vi "Trim Context.vi"(1 "Qualified Name":string) -> (0 "Name":string)   [LabVIEW 2020, in "Main.lvclass"]
uses:
  Main.lvclass
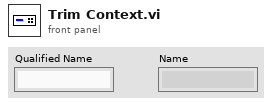
[diagram p1: front panel]
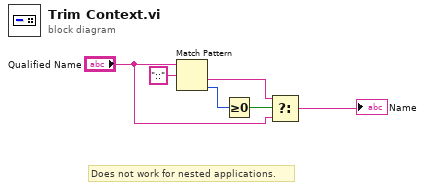
[diagram p0: block diagram]
diagram:
  # "Does not work for nested applications."
  n1 = Match Pattern(string="Qualified Name", regular expression="::") -> (after substring=w3:string, offset past match=w5:i32)  [unwired: 1 in, 2 out]
  n2 = Greater Or Equal To 0?(x=w5) -> (x >= 0?=w4:bool)
  n3 = Select(t=w3, s=w4, f="Qualified Name") -> (s? t:f=→"Name":string)
